vi "Record_to_TDMS.vi"() -> ()   [LabVIEW 2019]
uses:
  SubVIs/TypeDefs/StateRecording.ctl
  <vilib>/DAQmx/read.llb/DAQmx Read (Analog 1D Wfm NChan NSamp).vi
  <vilib>/DAQmx/create/channels.llb/DAQmx Create Channel (AI-Voltage-Basic).vi
  <vilib>/DAQmx/configure/timing.llb/DAQmx Timing (Sample Clock).vi
  <vilib>/DAQmx/miscellaneous.llb/DAQmx Fill In Error Info.vi
  <vilib>/measure/madcrms.llb/Basic Averaged DC-RMS for 1 Chan.vi
  <vilib>/express/express analysis/Spectral/Block/exnSpectralBlock spectral measurements RMS poly.vi
  <vilib>/express/express analysis/Spectral/Block/exnSpectralBlock spectral measurements RMS WFM.vi
  <vilib>/express/express analysis/Spectral/XNode/ExpressSpectralMeasurementsBlockNode.xnode
  <vilib>/measure/NI_MAPro.lvlib
panel:
  out "Time":u8(slide) scale=0.0..15.0
  out "Recordings":u8(slide) scale=0.0..50.0
  in  "stop":bool
  in  "Pause time [s]":dbl=15.0 caption="Time Target (s)"
  out "State":string
  in  "Record":bool
  out "Waveform":waveform(dbl)[](graph)
  out "Spectrum":cluster{"f0":dbl, "df":dbl, "magnitude":dbl[]}(graph)
  in  "sample rate":dbl=10000.0 format="%#_13g"
  in  "samples per channel":i32=10000
  in  "Filename":string
  in  "Recording time [s]":dbl=15.0 caption="Time Target (s)"
  in  "Number of recordings":i32
  in  "Recording directory":path
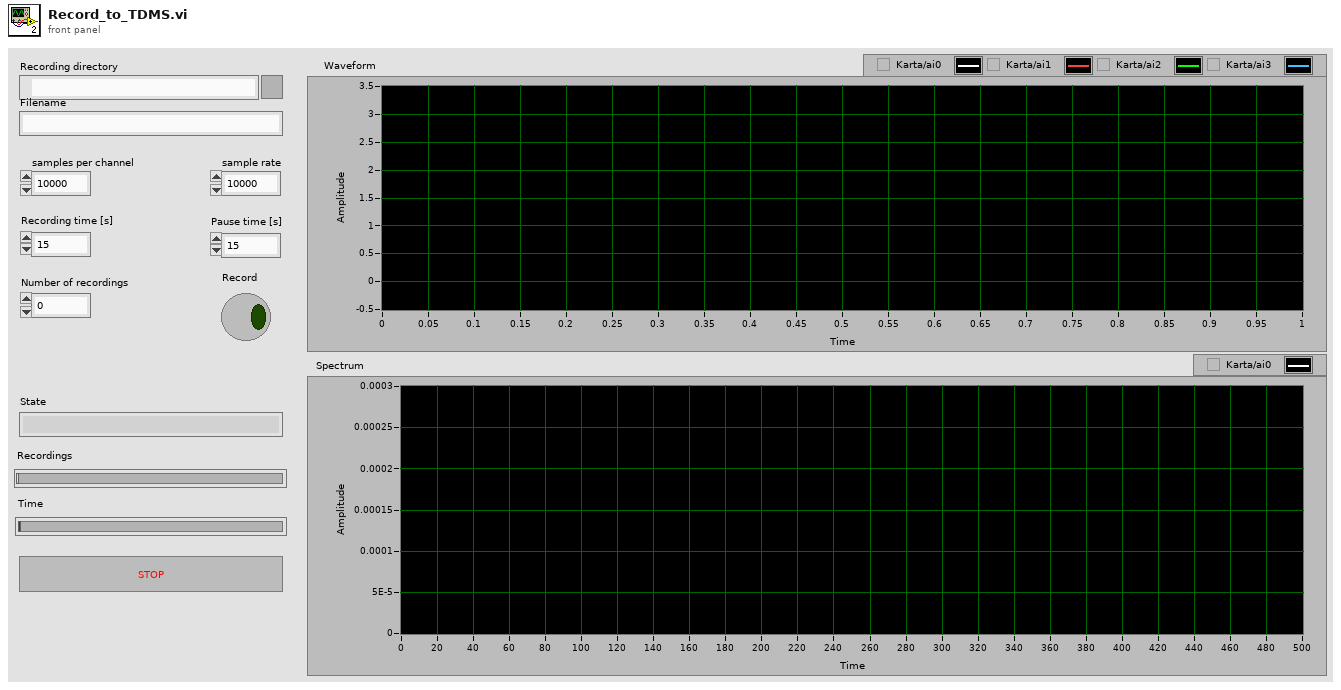
[diagram p1: front panel]
types:
  T1 = typedef "StateRecording.ctl" = enum16{"IDLE", "RECORDING", "PAUSE"}
  T2 = enum16{"open", "open or create", "create or replace", "create", "open (read-only)"}
  T3 = cluster{"averaging mode":u16, "weighting mode":u16, "number of averages":u32}
  T4 = cluster{"dB On (F)":bool, "unwrap phase (F)":bool, "convert to degree (F)":bool}
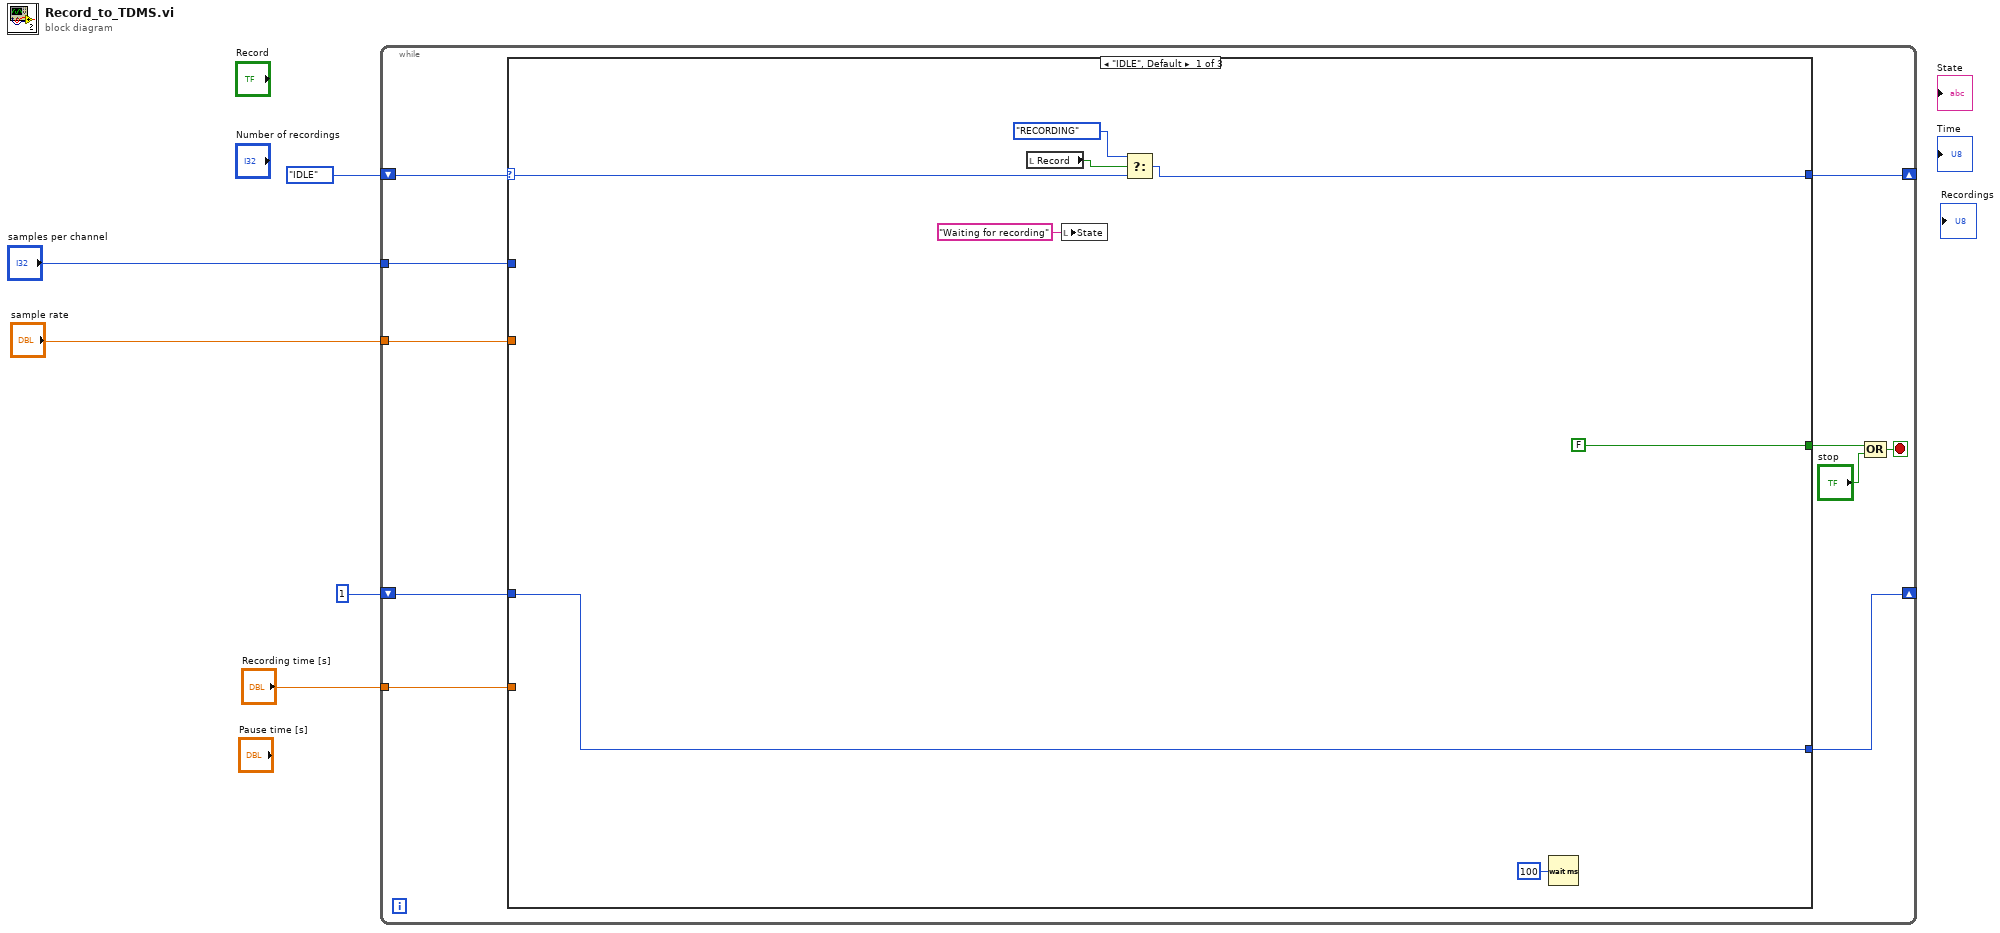
[diagram p0: block diagram]
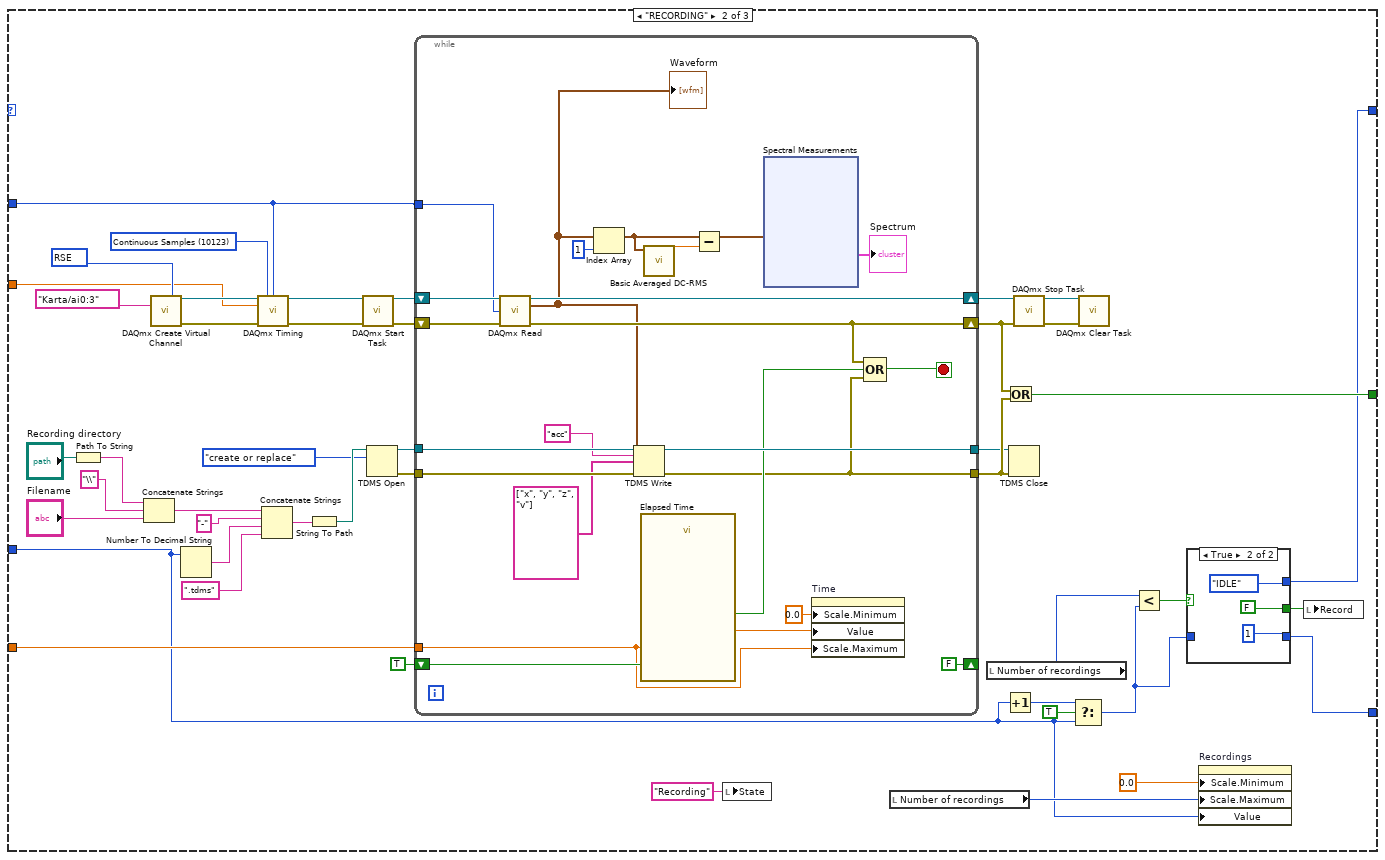
[diagram p2: hidden frame]
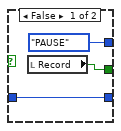
[diagram p3: hidden frame]
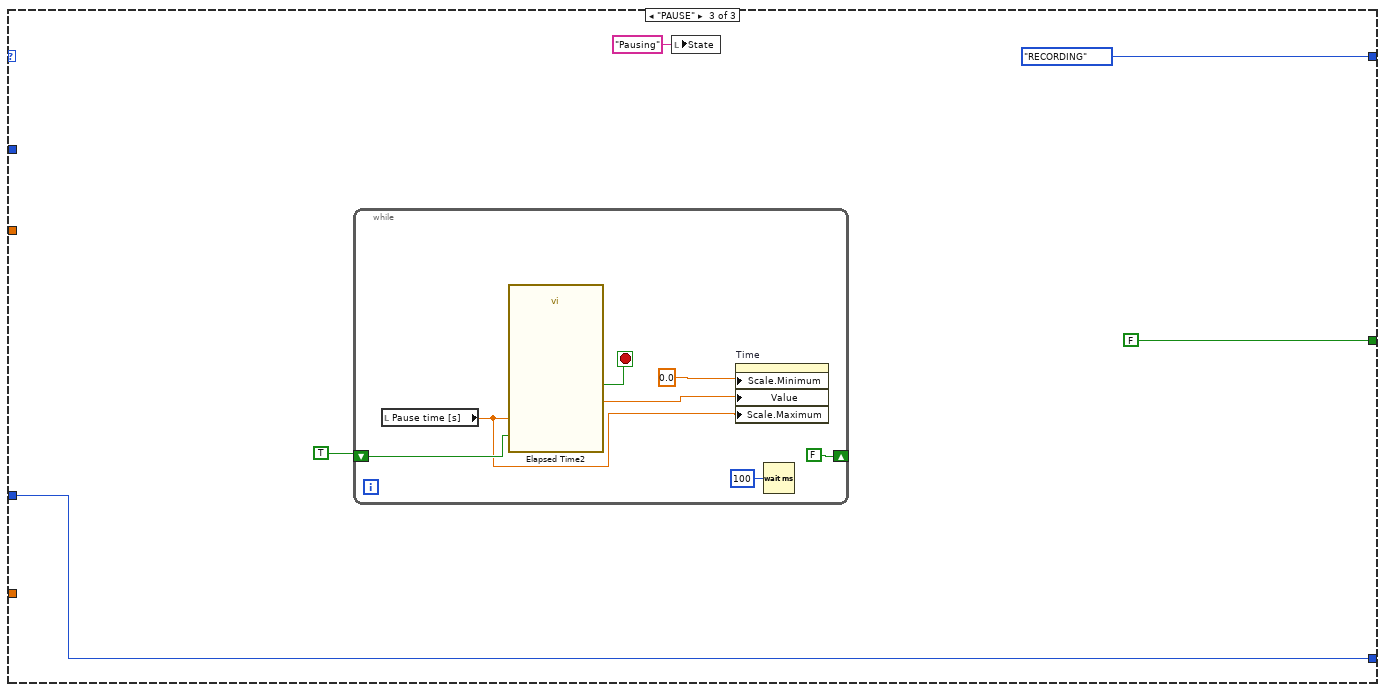
[diagram p4: hidden frame]
diagram:
  n1 = while {
    tunnel: "Recording time [s]" -> [w15]
    shift-right: [w11] -> _
    shift-left: 1 -> [w14]
    shift-right: [w12] -> _
    shift-left: StateRecording."IDLE" -> [w13]
    tunnel: "samples per channel" -> [w8]
    tunnel: "sample rate" -> [w7]
    stop <- w10 stop-if-true
    n2 = case shown="\"IDLE\", Default" w13 {
      selector: w13 -> [w22 _ _]
      tunnel: w15 -> [_ w57 _]
      tunnel: w14 -> [w23 w30 w113]
      tunnel: [w23 w33 w113] -> w11
      tunnel: [w19 w36 StateRecording."RECORDING"] -> w12
      tunnel: [FALSE w51 FALSE] -> w9
      tunnel: w8 -> [_ w45 _]
      tunnel: w7 -> [_ w44 _]
      frame "IDLE", Default {
        n3 = local read "Record"() -> (w21:bool)
        n4 = local write "State"("Waiting for recording" ("State")) -> ()
        n5 = Select(t=StateRecording."RECORDING", s=w21, f=w22) -> (s? t:f=w19:T1)
        n6 = Wait (ms)(milliseconds to wait=u32 100) -> ()  [unwired: 1 out]
      }
      frame "RECORDING" {
        w47 = 10083 items=["Default"=-1, "RSE"=10083, "NRSE"=10078, "Differential"=10106, "Pseudodifferential"=12529] ("input terminal configuration")
        w48 = 10123 items=["Finite Samples"=10178, "Continuous Samples"=10123, "Hardware Timed Single Point"=12522] ("sample mode")
        n7 = Path To String(path="Recording directory") -> (string=w27:string)
        n8 = Concatenate Strings(w27, "\\" ("string"), "Filename") -> (w24:string)
        n9 = call-poly <vilib>:"DAQmx Create Virtual Channel.vi"("input terminal configuration"=w47, "physical channels"=tag "Karta/ai0:3") -> ("task out"=w49:refnum<k21>, "error out"=w50:errorcluster)  [unwired: 12 in]
        n10 = Number To Decimal String(number=w30) -> (decimal integer string=w66:string)  [unwired: 1 in]
        n11 = call-poly <vilib>:"DAQmx Timing.vi"("task/channels in"=w49, "sample mode"=w48, "samples per channel"=w45, "rate"=w44, "error in"=w50) -> ("task out"=w43:refnum<k21>, "error out"=w42:errorcluster)  [unwired: 9 in]
        n12 = Concatenate Strings(w24, "-" ("string"), w66, ".tdms" ("string")) -> (w67:string)
        n13 = String To Path(string=w67) -> (path=w68:path)
        n14 = call <vilib>:"DAQmx Start Task.vi"("task/channels in"=w43, "error in"=w42) -> ("task out"=w61:refnum<k21>, "error out"=w62:errorcluster)  [unwired: 12 in]
        n15 = TDMS Open(10:T2."create or replace" ("operation (0:open)"), 11:w68) -> (0:w65:errorcluster, 3:w64:refnum<k34>)  [unwired: 5 in]
        n16 = while {
          tunnel: w64 -> [w94]
          tunnel: w65 -> [w95]
          tunnel: [w93] -> w54
          tunnel: [w75] -> w56
          shift-right: [w96] -> w63
          shift-left: w61 -> [w98]
          shift-right: [w91] -> w55
          shift-left: w62 -> [w97]
          tunnel: w57 -> [w77]
          tunnel: w45 -> [w90]
          shift-right: [FALSE] -> _
          shift-left: TRUE -> [w80]
          stop <- w92 stop-if-true
          n17 = call-poly <vilib>:"DAQmx Read.vi"("task/channels in"=w98, "number of samples per channel"=w90, "error in"=w97) -> ("task out"=w96:refnum<k21>, "data"=w85:waveform(dbl)[], "error out"=w91:errorcluster)  [unwired: 10 in]
          "Waveform" <- w85
          n18 = Index Array(array=w85, index=1) -> (element=w83:waveform(dbl))
          n19 = TDMS Write(0:w94, 5:"acc" ("group name in (Untitled)"), 7:string[] ["x", "y", "z", "v"] ("channel name(s) in (Untitled)"), 9:w85, 11:w95) -> (4:w93:refnum<k34>, 15:w75:errorcluster)  [unwired: 1 in, 2 out]
          n20 = call "Elapsed Time"("Time Target (s)"=w77, "Reset"=w80) -> ("Elapsed Time (s)"=w76:dbl, "Time has Elapsed"=w89:bool)  [unwired: 10 in, 6 out]
          n21 = call-poly <vilib>:"Basic Averaged DC-RMS.vi"("signal in"=w83) -> ("DC value"=w81:dbl)  [unwired: 7 in, 3 out]
          n22 = Subtract(x=w83, y=w81) -> (x-y=w82:waveform(dbl))
          n23 = xnode "Spectral Measurements"("Signals"=w82) -> ("FFT - (RMS)"=→"Spectrum":cluster{"f0":dbl, "df":dbl, "magnitude":dbl[]})  [unwired: 1 in, 2 out]
          n24 = property on="Time" class="Slide (strict)"("Scale.Minimum"=0.0 ("Scale.Range:Minimum"), "Value"=w76, "Scale.Maximum"=w77) -> ()  [unwired: 2 in, 2 out]
          n25 = Compound Arithmetic op=OR(w91, w89, w75) -> (w92:bool)
        }
        n26 = local write "State"("Recording" ("State")) -> ()
        n27 = local read "Number of recordings"() -> (w31:i32)
        n28 = local read "Number of recordings"() -> (w38:i32)
        n29 = Increment(x=w30) -> (x+1=w53:i32)
        n30 = Or(x=w55, y=w56) -> (x .or. y?=w51:bool)
        n31 = TDMS Close(8:w56, 11:w54) -> ()  [unwired: 2 out]
        n32 = call <vilib>:"DAQmx Stop Task.vi"("task/channels in"=w63, "error in"=w55) -> ("task out"=w41:refnum<k21>, "error out"=w40:errorcluster)  [unwired: 12 in]
        n33 = Select(t=w53, s=TRUE, f=w30) -> (s? t:f=w34:i32)
        n34 = call <vilib>:"DAQmx Clear Task.vi"("task in"=w41, "error in"=w40) -> ()  [unwired: 13 in, 1 out]
        n35 = Less?(x=w38, y=w34) -> (x < y?=w37:bool)
        n36 = case shown="True" w37 {
          tunnel: w34 -> [w71 _]
          tunnel: [w71 1] -> w33
          tunnel: [StateRecording."PAUSE" StateRecording."IDLE"] -> w36
          tunnel: [w69 FALSE ("t")] -> w35
          frame False {
            n37 = local read "Record"() -> (w69:bool)
          }
          frame True {
          }
        }
        n38 = property on="Recordings" class="Slide (strict)"("Scale.Minimum"=0.0 ("Scale.Range:Minimum"), "Scale.Maximum"=w31, "Value"=w30) -> ()  [unwired: 2 in, 2 out]
        n39 = local write "Record"(w35) -> ()
      }
      frame "PAUSE" {
        n40 = while {
          shift-right: [FALSE] -> _
          shift-left: TRUE -> [w118]
          stop <- w119 stop-if-true
          n41 = local read "Pause time [s]"() -> (w114:dbl)
          n42 = call "Elapsed Time2"("Time Target (s)"=w114, "Reset"=w118) -> ("Elapsed Time (s)"=w116:dbl, "Time has Elapsed"=w119:bool)  [unwired: 10 in, 6 out]
          n43 = property on="Time" class="Slide (strict)"("Scale.Minimum"=0.0 ("Scale.Range:Minimum"), "Value"=w116, "Scale.Maximum"=w114) -> ()  [unwired: 2 in, 2 out]
          n44 = Wait (ms)(milliseconds to wait=u32 100) -> ()  [unwired: 1 out]
        }
        n45 = local write "State"("Pausing" ("State")) -> ()
      }
    }
    n46 = Compound Arithmetic op=OR(w9, "stop") -> (w10:bool)
  }
